vi "RSZVB Get Power Port Limit State.vi"(8 "error in (no error)":errorcluster {"code" format="%.0x"}, 9 "Port (1)":i32=1, 10 "Channel (1)":i32=1, 11 "VISA session":refnum<visa-resource-name>) -> (0 "error out":errorcluster {"code" format="%.0x"}, 2 "Limit State":bool, 3 "dup VISA session":refnum<visa-resource-name>)   [LabVIEW 2011]
doc: "Queries the state of the limit for the source power at port no. <Pt>.\n\nRemote-control command(s):\nSOURce<Ch>:POWer<Pt>[:LEVel][:IMMediate]LLIMit[:STATe]?"
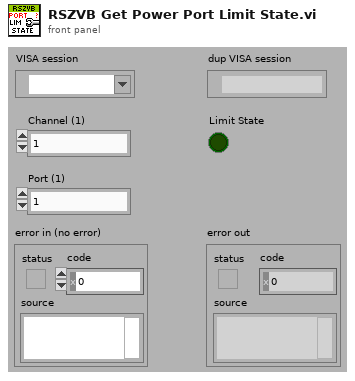
[diagram p1: front panel]
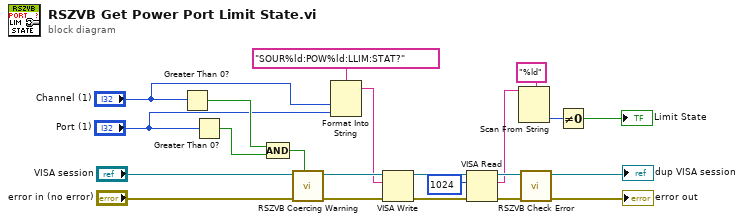
[diagram p0: block diagram]
diagram:
  n1 = Greater Than 0?(x="Channel (1)") -> (x > 0?=w9:bool)
  n2 = Greater Than 0?(x="Port (1)") -> (x > 0?=w10:bool)
  n3 = Compound Arithmetic op=AND(w9, w10) -> (w6:bool)
  n4 = call "RSZVB Coercing Warning.vi"("In Range?"=w6, "error in (no error)"="error in (no error)", "VISA session"="VISA session") -> ("error out"=w20:errorcluster, "dup VISA session"=w21:refnum<visa-resource-name>)  [unwired: 7 in]
  n5 = Format Into String(format string="SOUR%ld:POW%ld:LLIM:STAT?", "Channel (1)", "Port (1)") -> (resulting string=w19:string)  [unwired: 2 in, 1 out]
  n6 = VISA Write(VISA resource name=w21, write buffer=w19, error in (no error)=w20) -> (VISA resource name out=w12:refnum<visa-resource-name>, error out=w11:errorcluster)  [unwired: 1 out]
  n7 = VISA Read(VISA resource name=w12, byte count=u32 1024 ("byte count (0)"), error in (no error)=w11) -> (VISA resource name out=w17:refnum<visa-resource-name>, read buffer=w14:string, error out=w16:errorcluster)  [unwired: 1 out]
  n8 = Scan From String(format string="%ld", input string=w14) -> (output 1=w13:i32)  [unwired: 3 in, 3 out]
  n9 = call "RSZVB Check Error.vi"("error in (no error)"=w16, "VISA session"=w17) -> ("error out"=→"error out":errorcluster, "dup VISA session"=→"dup VISA session":refnum<visa-resource-name>)  [unwired: 8 in]
  n10 = Not Equal To 0?(x=w13) -> (x != 0?=→"Limit State":bool)
